vi "ST Const.vi"() -> (0 "Robot Constants":cluster{i32[], i32[], dbl[]})   [LabVIEW 2009]
doc: "This VI supplies constants associated with the actual R17 Robot. They are:\nThe lengths in mm of each \"arm\"\nThe gear ratio, the number of motor steps in 90 degrees\nThe limits of motion from the home position in radians +/-\n\nThe input values are for a gripper to be attached by the user."
panel:
  out "Motion Limits":dbl[](array[numeric])
  in  "Limits":i32
  out "Gear Ratios":i32[](array[numeric])
  in  "Gear Ratio":i32
  out "Arm Lengths":i32[](array[numeric])
  in  "Arm Length":i32=50
  # "Constants for the R17 Robot"
  # "Gripper Values"
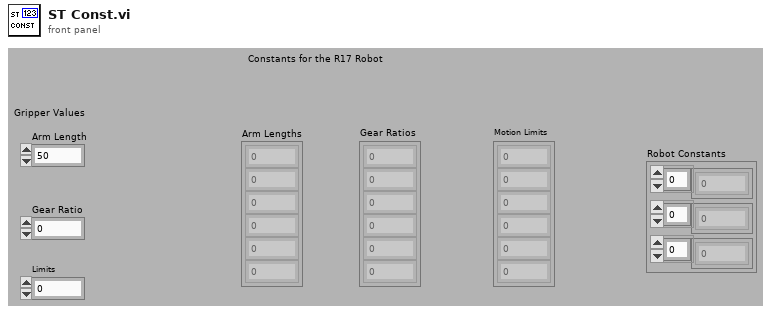
[diagram p1: front panel]
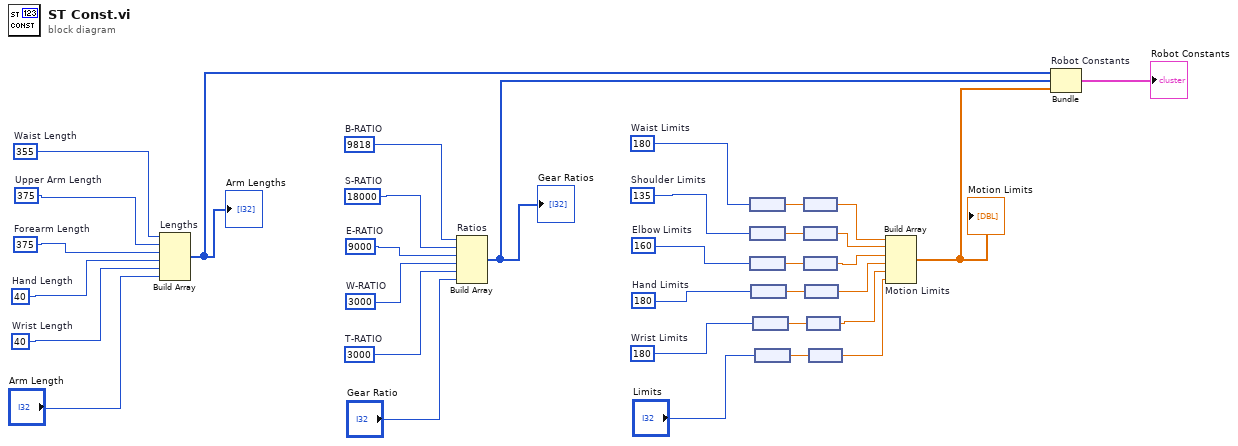
[diagram p0: block diagram]
diagram:
  w12 = 180  # Wrist Limits
  w10 = 180  # Hand Limits
  w9 = 160  # Elbow Limits
  w18 = 135  # Shoulder Limits
  w21 = 180  # Waist Limits
  w24 = 3000  # T-RATIO
  w25 = 3000  # W-RATIO
  w26 = 9000  # E-RATIO
  w27 = 18000  # S-RATIO
  w28 = 9818  # B-RATIO
  w30 = 40  # Wrist Length
  w31 = 40  # Hand Length
  w32 = 375  # Forearm Length
  w33 = 375  # Upper Arm Length
  w34 = 355  # Waist Length
  n1 = Build Array "Lengths"(w34, w33, w32, w31, w30, "Arm Length") -> (w2:i32[])
  "Arm Lengths" <- w2
  n2 = Build Array "Ratios"(w28, w27, w26, w25, w24, "Gear Ratio") -> (w3:i32[])
  "Gear Ratios" <- w3
  n3 = node(w21) -> (w22:dbl[unit])
  n4 = node(w18) -> (w19:dbl[unit])
  n5 = node(w9) -> (w16:dbl[unit])
  n6 = node(w10) -> (w15:dbl[unit])
  n7 = node(w12) -> (w14:dbl[unit])
  n8 = node("Limits") -> (w13:dbl[unit])
  n9 = node ("Convert Unit")(w22) -> (w20:dbl)
  n10 = node(w19) -> (w17:dbl)
  n11 = node(w16) -> (w8:dbl)
  n12 = node(w15) -> (w7:dbl)
  n13 = node(w14) -> (w6:dbl)
  n14 = node ("Radians")(w13) -> (w5:dbl)
  n15 = Build Array "Motion Limits"(w20, w17, w8, w7, w6, w5) -> (w4:dbl[])
  "Motion Limits" <- w4
  n16 = Bundle "Robot Constants"(w2, w3, w4) -> (→"Robot Constants":cluster{i32[], i32[], dbl[]})  [unwired: 1 in]
